vi "XL320_Write Word Over 2 Addresses.vi"(0 "VISA resource name":refnum<visa-resource-name>, 5 "Motor ID (0)":u8, 7 "Address number (0)":u16, 9 "Parameter (0)":u16, 11 "error in (no error)":errorcluster) -> (4 "VISA resource name out":refnum<visa-resource-name>, 15 "error out":errorcluster)   [LabVIEW 2017, in "Dynamixel XL320.lvlib"]
doc: "Writes a word type (U16) over two addresses in the motor's register. The data is written in little endian byte order. This is a Low-Level VI that is used by other VIs."
uses:
  <instrlib>/Dynamixel XL320 (Drivers instrument)/Dynamixel XL320.lvlib
  <instrlib>/Dynamixel XL320 (Drivers instrument)/Public/Configure/XL320_Select_Action.ctl
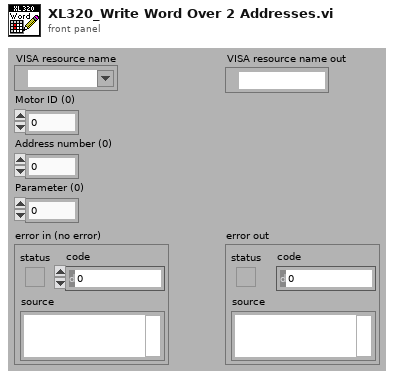
[diagram p1: front panel]
types:
  T1 = enum16{"big-endian, network order", "native, host order", "little-endian"}
  T2 = typedef "Dynamixel XL320.lvlib/XL320_Select_Action.ctl" = u8
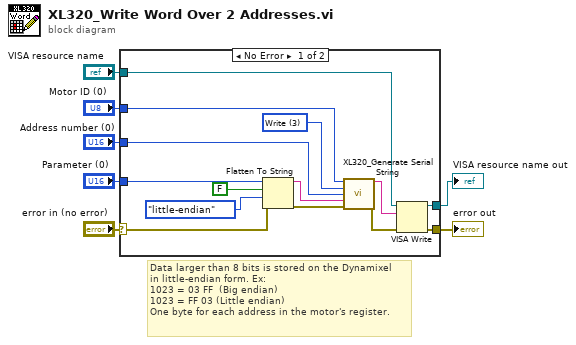
[diagram p0: block diagram]
diagram:
  # "Data larger than 8 bits is stored on the Dynamixel \nin little-endian form. Ex:\n1023 = 03 FF  (Big endian)\n1023 = FF 03 (Little endian)\nOne byte for each address in the motor's register."
  n1 = case shown="No Error" "error in (no error)" {
    selector: "error in (no error)" -> [w15 w23]
    tunnel: "Address number (0)" -> [w10 _]
    tunnel: "Motor ID (0)" -> [w9 _]
    tunnel: "VISA resource name" -> [w21 w22]
    tunnel: "Parameter (0)" -> [w18 _]
    tunnel: [w20 w22] -> w3
    tunnel: [w19 w23] -> w2
    frame No Error {
      w8 = T2 3 items=["Ping"=1, "Read"=2, "Write"=3, "Registered Write"=4, "Action"=5, "Reset"=6, "Reboot"=8, "Status"=85, "Sync Read"=130, "Sync Write"=131, "Bulk Read"=146, "Bulk Write"=147] ("Select Action")
      n2 = Flatten To String(anything=w18, prepend array or string size? (T)=FALSE, byte order (0:big-endian, network order)=T1."little-endian", error in (no error)=w15) -> (data string=w11:string, error out=w12:errorcluster)  [unwired: 1 out]
      n3 = call <instrlib>:"XL320_Generate Serial String.vi"("Motor ID"=w9, "Select Action"=w8, "Address"=w10, "Parameters"=w11, "Error in (no error)"=w12) -> ("Command to Serial"=w14:string, "error out"=w13:errorcluster)  [unwired: 9 in]
      n4 = VISA Write(VISA resource name=w21, write buffer=w14, error in (no error)=w13) -> (VISA resource name out=w20:refnum<visa-resource-name>, error out=w19:errorcluster)  [unwired: 1 out]
    }
    frame Error {
    }
  }
  "VISA resource name out" <- w3
  "error out" <- w2
